vi "FrequencyCounterStart.vi"(0 "Device Info":T1={"Serial Number"=-1, "Channel"=0, "Port"=0}, 1 "Filter Type":u32(ring)=1 items=["FILTER_TYPE_ZERO_CROSSING"=1, "FILTER_TYPE_LOGIC_LEVEL"=2], 2 "FrequencyCutoff":dbl=1.0, 3 "DataInterval":i32=-1, 5 "Power Supply":i32(ring)=2 items=["POWER_SUPPLY_OFF"=1, "POWER_SUPPLY_12V"=2, "POWER_SUPPLY_24V"=3], 7 "Input Mode":i32(ring)=1 items=["INPUT_MODE_NPN"=1, "INPUT_MODE_PNP"=2], 11 "error in (no error)":errorcluster, 12 "Connection":u16(ring) items=["No Preference", "Remote", "Local"], 13 "Timeout (mSec)":i32=5000) -> (4 "Phidget ID":u64, 6 "Serial Number Return":i32, 10 "Attached?":bool, 15 "error out":errorcluster)   [LabVIEW 2012, in "Phidget Frequency Counter.lvlib"]
doc: "${FrequencyCounter:StartHeader}"
uses:
  <instrlib>/Phidgets/Phidget Frequency Counter/Phidget Frequency Counter.lvlib
  <instrlib>/Phidgets/Phidget Common/Phidget Common.lvlib
  <instrlib>/Phidgets/Phidget Encoder/Phidget Encoder.lvlib
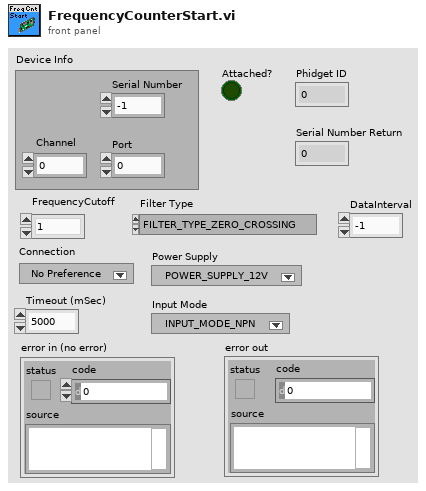
[diagram p1: front panel]
types:
  T1 = cluster{"Serial Number":i32, "Channel":i32, "Port":i32}
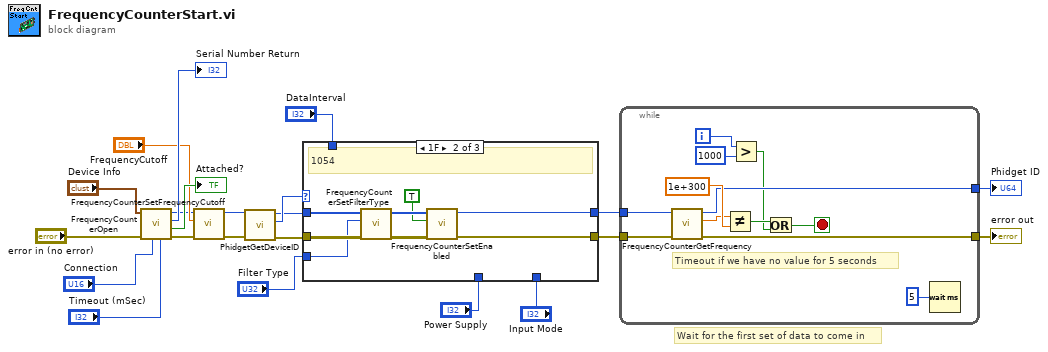
[diagram p0: block diagram]
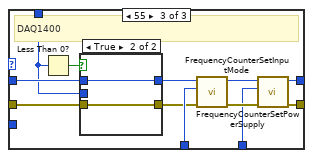
[diagram p3: hidden frame]
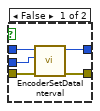
[diagram p4: hidden frame]
diagram:
  # "Wait for the first set of data to come in"
  n1 = call <instrlib>:"FrequencyCounterOpen.vi"("Timeout (mSec)"="Timeout (mSec)", "Connection"="Connection", "error in"="error in (no error)", "Device Info"="Device Info") -> ("error out"=w11:errorcluster, "Attached?"=→"Attached?":bool, "Serial Number Return"=→"Serial Number Return":i32, "Phidget ID"=w12:u64)  [unwired: 4 in]
  n2 = call <instrlib>:"FrequencyCounterSetFrequencyCutoff.vi"("error in (no error)"=w11, "FrequencyCutoff"="FrequencyCutoff", "Device In"=w12) -> ("error out"=w9:errorcluster, "Device Out"=w10:u64)  [unwired: 6 in]
  n3 = call <instrlib>:"PhidgetGetDeviceID.vi"("error in (no error)"=w9, "Device In"=w10) -> ("error out"=w6:errorcluster, "Devie IDs"=w8:u32, "Device Out"=w7:u64)  [unwired: 6 in]
  n4 = case shown="1F" w8 {
    tunnel: "Filter Type" -> [_ w30 _]
    tunnel: w6 -> [w23 w32 w36]
    tunnel: w7 -> [w24 w31 w37]
    tunnel: [w24 w25 w41] -> w5
    tunnel: [w23 w27 w42] -> w4
    tunnel: "Power Supply" -> [_ _ w40]
    tunnel: "Input Mode" -> [_ _ w39]
    tunnel: "DataInterval" -> [_ _ w35]
    frame 0, Default {
    }
    frame 31 {
      # "1054"
      n5 = call <instrlib>:"FrequencyCounterSetFilterType.vi"("error in (no error)"=w32, "Filter Type"=w30, "Device In"=w31) -> ("error out"=w28:errorcluster, "Device Out"=w26:u64)  [unwired: 6 in]
      n6 = call <instrlib>:"FrequencyCounterSetEnabled.vi"("error in (no error)"=w28, "Enabled"=TRUE, "Device In"=w26) -> ("error out"=w27:errorcluster, "Device Out"=w25:u64)  [unwired: 6 in]
    }
    frame 55 {
      # "DAQ1400"
      n7 = Less Than 0?(x=w35) -> (x < 0?=w38:bool)
      n8 = case shown="True" w38 {
        tunnel: w37 -> [w48 w51]
        tunnel: w36 -> [w49 w50]
        tunnel: [w47 w51] -> w34
        tunnel: [w46 w50] -> w33
        tunnel: w35 -> [w45 _]
        frame False {
          n9 = call <instrlib>:"EncoderSetDataInterval.vi"("error in (no error)"=w49, "Interval"=w45, "Device In"=w48) -> ("error out"=w46:errorcluster, "Device Out"=w47:u64)  [unwired: 6 in]
        }
        frame True {
        }
      }
      n10 = call <instrlib>:"FrequencyCounterSetPowerSupply.vi"("error in (no error)"=w33, "Power Supply"=w40, "Device In"=w34) -> ("error out"=w43:errorcluster, "Device Out"=w44:u64)  [unwired: 6 in]
      n11 = call <instrlib>:"FrequencyCounterSetInputMode.vi"("error in (no error)"=w43, "Input Mode"=w39, "Device In"=w44) -> ("error out"=w42:errorcluster, "Device Out"=w41:u64)  [unwired: 6 in]
    }
  }
  n12 = while {
    tunnel: w5 -> [w61]
    tunnel: w4 -> [w60]
    tunnel: [w58] -> w19
    tunnel: [w59] -> w21
    i -> [w56]
    stop <- w53 stop-if-true
    # "Timeout if we have no value for 5 seconds"
    n13 = call <instrlib>:"FrequencyCounterGetFrequency.vi"("error in (no error)"=w60, "Device In"=w61) -> ("error out"=w59:errorcluster, "Frequency"=w52:dbl, "Device Out"=w58:u64)  [unwired: 6 in]
    n14 = Not Equal?(x=w52, y=1e+300) -> (x != y?=w55:bool)
    n15 = Greater?(x=w56, y=1000) -> (0:w54:bool)
    n16 = Or(x=w55, y=w54) -> (x .or. y?=w53:bool)
    n17 = Wait (ms)(milliseconds to wait=u32 5) -> ()  [unwired: 1 out]
  }
  "error out" <- w21
  "Phidget ID" <- w19
